vi "AddManySingle.vi"(7 "Priority":refnum<class "Action.lvclass">[](array[class]), 10 "Standard":refnum<class "Action.lvclass">, 11 "Stack in":refnum<class "Stack.lvclass">) -> (3 "Stack out":refnum<class "Stack.lvclass">)   [LabVIEW 2024, in "ActionStack.lvlib" / "Stack.lvclass"]
uses:
  Stack.lvclass
  Action/Action.lvclass
  Stack.lvclass/Stack.ctl
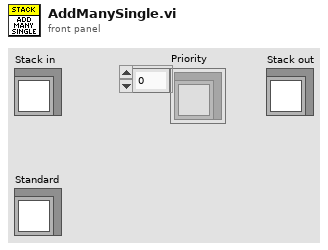
[diagram p1: front panel]
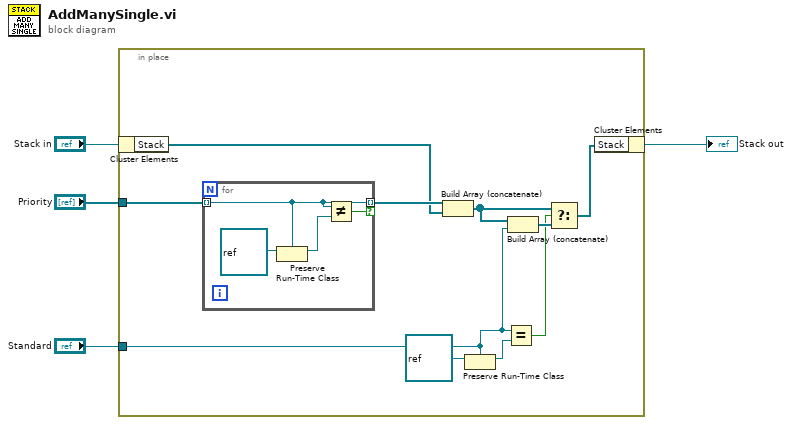
[diagram p0: block diagram]
diagram:
  n1 = in-place {
    in-place-border: "Priority" -> [w12]
    in-place-border: "Standard" -> [w11]
    n2 = in-place-cluster #1("Stack in") -> ("Stack"=w6:refnum<class "Action.lvclass">[])
    n3 = for {
      tunnel: w12 -> [w16] mode=indexing
      tunnel: [w16] -> w8 mode=indexing if=w15
      n4 = Preserve Run-Time Class(object in=refnum<class> refnum, 2:w16) -> (object out=w17:refnum<class "Action.lvclass">)  [unwired: 1 in, 1 out]
      n5 = Not Equal?(x=w16, y=w17) -> (x != y?=w15:bool)
    }
    n6 = Build Array (concatenate)(w8, w6) -> (w7:refnum<class "Action.lvclass">[])
    n7 = Preserve Run-Time Class(object in=refnum<class> refnum, 2:w11) -> (object out=w13:refnum<class "Action.lvclass">)  [unwired: 1 in, 1 out]
    n8 = Equal?(x=w11, y=w13) -> (x = y?=w9:bool)
    n9 = Build Array (concatenate)(w7, w11) -> (w10:refnum<class "Action.lvclass">[])
    n10 = Select(t=w7, s=w9, f=w10) -> (s? t:f=w5:refnum<class "Action.lvclass">[])
    n11 = in-place-cluster #1("Stack"=w5) -> (→"Stack out":refnum<class "Stack.lvclass">)
  }
